vi "DSF.Execution.Builder.Set VS Channel Buffer.vi"(8 "error in (no error)":errorcluster, 10 "VS Channel Buffer":dbl[](array[numeric]), 11 "Builder in":refnum<class "DSF.Execution.Builder.lvclass">) -> (0 "error out":errorcluster, 3 "Builder out":refnum<class "DSF.Execution.Builder.lvclass">)   [LabVIEW 2016, in "DSF.Engine.lvlib" / "DSF.Execution.Builder.lvclass"]
uses:
  DSF.Execution.Builder.lvclass
  DSF.Execution.Builder.lvclass/DSF.Execution.Builder.ctl
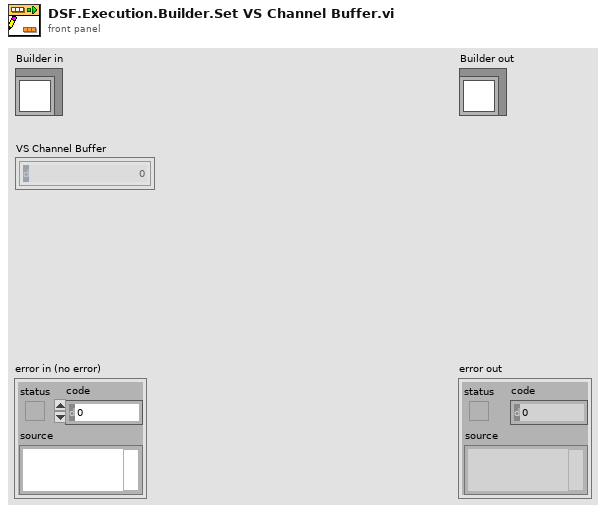
[diagram p1: front panel]
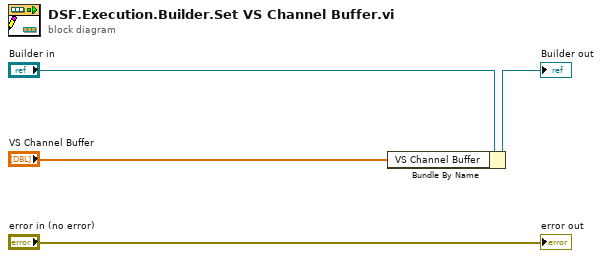
[diagram p0: block diagram]
diagram:
  n1 = Bundle By Name(cluster="Builder in", "VS Channel Buffer"="VS Channel Buffer") -> (→"Builder out":refnum<class "DSF.Execution.Builder.lvclass">)
  "error out" <- "error in (no error)"
